vi "auto_save_settings.vi"(8 "error in":errorcluster, 10 "base path":path, 11 "all settings":T1={"Variable Settings"={"Measurement Timeout (ms)"=0}, "HSDIO Settings"={"Enable HSDIO Pulses"=TRUE, "Resource Name"="PXI1Slot6", "Clock Rate"=20000000.0, "Array of Script Triggers"=[], "Pulse Generation Script"="script script1\n     Generate RedTrap_compress_temp\nend script", "Start Trigger"={"Wait for start trigger?"=FALSE, "source (PFI 0)"="PFI0", "edge (rising)"=12, "description"=""}, "Hardware alignment quantum\n(in samples)"=1, "Inital State"="", "Idle State"="", "Active Channels"="", "Array of Waveforms"=[], "description"=""}, "DAQmx Pulse Settings"={"Enable DAQmx Pulses"=FALSE, "DAQmx Physical Channels"="", "Clock Rate"=0.0, "units/sec (ms=1000)"=0.0, "Start Trigger"={"Wait for start trigger?"=FALSE, "source"="", "edge"=0}, "Timing Sequence Control"=[]}, "DDS Settings"={"Enable DDS"=FALSE, "Array of DDS Boxes"=[]}, "Camera settings"={"Analog Gain (0-5)"=4, "Exposure Time"=0.01, "EM Gain (0-255)"=0, "Trigger Polarity"="ATP P", "External Trigger Mode"="EMD E", "Scan Speed"="SSP H", "External Trigger Source"="ESC B", "Scan Mode"="SMD N", "Super Pixel Binning\n(if enabled in Scan Mode)"="SPX 1", "Camera Sub-array acquisition region\n(if enabled in scan mode)"={"Left"=0, "Top"=0, "Width"=0, "Height"=0}, "Use camera?"=FALSE, "# image buffers"=100, "shots per measurement"=100, "Force images to U16"=FALSE, "Low Light Sensitivity"="LLS 0", "cooling"="CSW F", "fan"="FAN F", "Frame Grabber acquisition region"={"Left"=0, "Top"=0, "Right"=0, "Bottom"=0}}, "Counter Settings"={"Enable Counters"=FALSE, "Array of Counter Settings"=[]}, "Filter Cluster"={"Counter Filter thresholds"=[], "Data Filters\nROI Minimum Thresholds"=[]}, "Analog Output Parameters"={"Enable Analog Out?"=FALSE, "Physical Channel"="PXI1Slot2/ao0:2", "Minimum Value"=-10.0, "Maximum Value"=10.0, "Samples per second"=0.0, "Total AO Time (seconds)"=0.0, "Start Trigger"={"Wait for start trigger?"=FALSE, "source"="/Dev1/PFI0", "edge"=10280}, "Analog Output Waveforms (channel, time)"=[], "Export trigger"={"Export Start Trigger?"=FALSE, "output terminal"=""}}, "Notes"="", "HP83623A Generator Settings Array"=[], "Iteration Graph Settings"={"Plot Regions"="", "Plot Shots"=""}, "PI Piezo Settings"={"Enable"=FALSE, "Array of Piezo Controllers"=[]}, "Andor settings"={"Andor Path"=path "", "Copy any Andor files"=FALSE, "Wait time before copying Andor files (ms)"=0}, "Measurement Chart Settings"={"Which regions to plot (comma separated)"="", "Which shot to plot"=0}, "HP8662A Synthesized Signal Generator Array"=[], "HP83712B Synthesized CW Generator Array"=[], "TTL input"={"Enable"=FALSE, "lines"=""}} {"HSDIO Settings"."Hardware alignment quantum\n(in samples)" min=1 step=1; "HSDIO Settings"."Array of Script Triggers"."level" items=["High Level"=34, "Low Level"=35]; "HSDIO Settings"."Array of Script Triggers"."edge" items=["Rising Edge"=12, "Falling Edge"=13]; "HSDIO Settings"."Start Trigger"."edge (rising)" items=["Rising Edge"=12, "Falling Edge"=13]; "HSDIO Settings"."Clock Rate" min=0.0 max=200000000.0 format="%.2p"; "DAQmx Pulse Settings"."Start Trigger"."edge" items=["Rising"=10280, "Falling"=10171]; "DAQmx Pulse Settings"."Clock Rate" min=0.0 max=200000000.0 format="%.2p"; "Camera settings"."Frame Grabber acquisition region"."Bottom" max=512 step=1; "Camera settings"."Frame Grabber acquisition region"."Right" max=512 step=1; "Camera settings"."Frame Grabber acquisition region"."Top" max=512 step=1; "Camera settings"."Frame Grabber acquisition region"."Left" max=512 step=1; "Camera settings"."shots per measurement" min=0 step=1; "Camera settings"."# image buffers" min=0 step=1; "Camera settings"."Camera Sub-array acquisition region\n(if enabled in scan mode)"."Height" min=16 max=512 step=16; "Camera settings"."Camera Sub-array acquisition region\n(if enabled in scan mode)"."Width" min=16 max=512 step=16; "Camera settings"."Camera Sub-array acquisition region\n(if enabled in scan mode)"."Top" max=496 step=16; "Camera settings"."Camera Sub-array acquisition region\n(if enabled in scan mode)"."Left" max=496 step=16; "Camera settings"."Analog Gain (0-5)" max=5 step=1; "Counter Settings"."Array of Counter Settings"."Binwidth (ms)" format="%0.2f"; "Analog Output Parameters"."Start Trigger"."edge" items=["Rising"=10280, "Falling"=10171]; "Analog Output Parameters"."Maximum Value" format="%0.2f"; "Analog Output Parameters"."Minimum Value" format="%0.2f"}) -> (0 "error out":errorcluster)   [LabVIEW 2013]
doc: "This .vi save all the experiment settings to autosave_settings.xml in the input directory, without any prompts. For use in autosaving all settings at the beginning of each experiment.\n\nMTL 2012 Dec 27"
uses:
  Analog_output/AO_settings.ctl
  Analog_output/Analog_Output.lvclass
  filters/filters.ctl
  Counter/Counter_Settings_Control.ctl
  Counter/Counter.lvclass
  Camera/Hamamatsu_C9100-13/camera_setup.ctl
  Camera/Hamamatsu_C9100-13/Hamamatsu_C9100-13.lvclass
  <vilib>/ni845x/ni845x.llb/ni845xControl.ctl
  DDS drivers v3/DDS_box_device_reference.ctl
  DDS drivers v3/DDS RAM mode.ctl
  DDS drivers v3/DDS_box_cluster.ctl
  DDS drivers v3/Array_of_DDS_Boxes.ctl
  DDS/DDS_Settings_Cluster.ctl
  DAQmx_pulse_out/settings.ctl
  DAQmx_pulse_out/DAQmx_pulse_out.lvclass
  <instrlib>/niHSDIO/niHSDIO.llb/niHSDIO_ctl Trigger Source Values (Ring).ctl
  <instrlib>/niHSDIO/niHSDIO.llb/niHSDIO_ctl Trigger DigEdge - Edge Values (Ring).ctl
  <instrlib>/niHSDIO/niHSDIO.llb/niHSDIO_ctl Trigger Script - trigID Values (Ring).ctl
  <instrlib>/niHSDIO/niHSDIO.llb/niHSDIO_ctl Trigger DigLvl - Level Values (Ring).ctl
  HSDIO/HSDIO_settings.ctl
  HSDIO/HSDIO.lvclass
  all_settings.ctl
  GPIB/HP83623A_RF_Generator/HP83623A_array.ctl
  GPIB/HP83623A_RF_Generator/HP83623A_RF_Generator.lvclass
  PI_piezo/settings.ctl
  PI_piezo/PI_Piezo.lvclass
  Camera/Andor/Andor_settings.ctl
  gui/measurement_graph.ctl
  GPIB/RF_Generator_settings.ctl
  GPIB/GPIB.lvclass
  GPIB/RF_Generator_settings_array.ctl
  DDS drivers v3/DDS_profile.ctl
  DDS drivers v3/DDS_channel.ctl
  DDS/DDS.lvclass
  DDS drivers v3/array_of_DDS_profiles.ctl
  DDS drivers v3/array_of_DDS_channels.ctl
  TTL_input/TTL_input_settings.ctl
  TTL_input/TTL_input.lvclass
  HSDIO/waveform.ctl
  PI_piezo/piezo_channel.ctl
  PI_piezo/piezo_controller.ctl
  GPIB/HP83623A_RF_Generator/HP83623A.ctl
  ExperimentVariables/Variable_Settings.ctl
panel:
  # "Regions of Interest -->"
  # "Shots\n   |\n  V"
  # "Counters -->"
  # "Counter\n    bins\n       |\n      V"
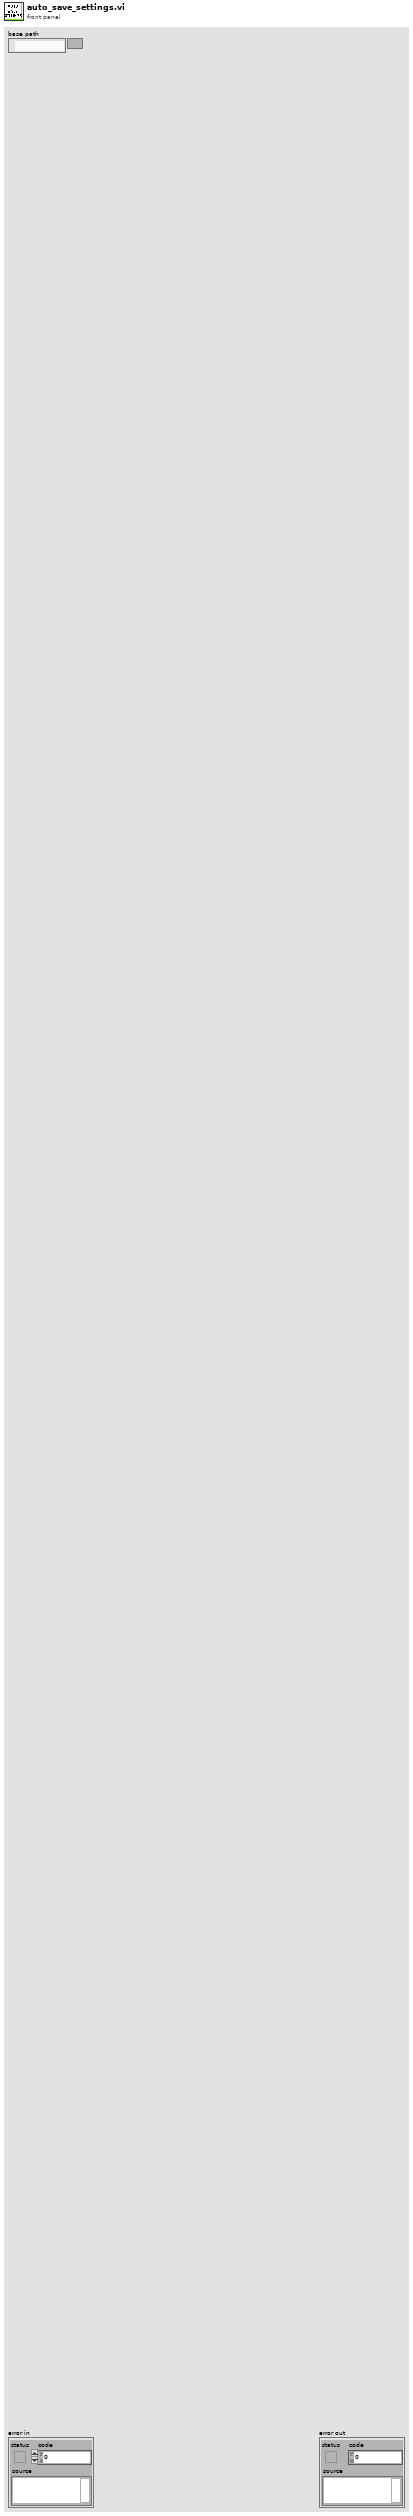
[diagram p1: front panel]
types:
  T1 = typedef "all_settings.ctl" = cluster{"Variable Settings":T2, "HSDIO Settings":T3, "DAQmx Pulse Settings":T9, "DDS Settings":T10, "Camera settings":T20, "Counter Settings":T21, "Filter Cluster":T22, "Analog Output Parameters":T23, "Notes":string, "HP83623A Generator Settings Array":T24, "Iteration Graph Settings":cluster{"Plot Regions":string, "Plot Shots":string}, "PI Piezo Settings":T26, "Andor settings":T29, "Measurement Chart Settings":T30, "HP8662A Synthesized Signal Generator Array":T31, "HP83712B Synthesized CW Generator Array":T31, "TTL input":T33}
  T2 = typedef "Variable_Settings.ctl" = cluster{"Measurement Timeout (ms)":u32}
  T3 = typedef "HSDIO.lvclass/HSDIO_settings.ctl" = cluster{"Enable HSDIO Pulses":bool, "Resource Name":refnum<k15>, "Clock Rate":dbl, "Array of Script Triggers":cluster{"trigger id (script trigger 0)":T4, "source (PFI 0)":T5, "Trigger Type":enum32{"Edge", "Level"}, "edge":T6, "level":T7}[], "Pulse Generation Script":string, "Start Trigger":cluster{"Wait for start trigger?":bool, "source (PFI 0)":T5, "edge (rising)":T6, "description":string}, "Hardware alignment quantum\n(in samples)":u16, "Inital State":string, "Idle State":string, "Active Channels":string, "Array of Waveforms":T8[], "description":string}
  T4 = typedef "niHSDIO_ctl Trigger Script - trigID Values (Ring).ctl" = string
  T5 = typedef "niHSDIO_ctl Trigger Source Values (Ring).ctl" = string
  T6 = typedef "niHSDIO_ctl Trigger DigEdge - Edge Values (Ring).ctl" = i32
  T7 = typedef "niHSDIO_ctl Trigger DigLvl - Level Values (Ring).ctl" = i32
  T8 = typedef "HSDIO.lvclass/waveform.ctl" = cluster{"name":string, "transitions":u32[], "states":u8[][]}
  T9 = typedef "DAQmx_pulse_out.lvclass/settings.ctl" = cluster{"Enable DAQmx Pulses":bool, "DAQmx Physical Channels":tag, "Clock Rate":dbl, "units/sec (ms=1000)":dbl, "Start Trigger":cluster{"Wait for start trigger?":bool, "source":tag, "edge":i32}, "Timing Sequence Control":string[][]}
  T10 = typedef "DDS_Settings_Cluster.ctl" = cluster{"Enable DDS":bool, "Array of DDS Boxes":T11}
  T11 = typedef "Array_of_DDS_Boxes.ctl" = T12[]
  T12 = typedef "DDS_box_cluster.ctl" = cluster{"DDS box device reference":T13, "Array of DDS Channels (4)":T15, "Enable":bool, "description":string}
  T13 = typedef "DDS_box_device_reference.ctl" = cluster{"NI USB-8451 device reference":T14, "DIO port":u8, "Serial Clock Rate [kHz]":u16}
  T14 = typedef "ni845xControl.ctl" = refnum<k21>
  T15 = typedef "DDS.lvclass/array_of_DDS_channels.ctl" = T16[]
  T16 = typedef "DDS.lvclass/DDS_channel.ctl" = cluster{"Power":bool, "Channel Parameters":cluster{"Ref Clock Rate [kHz]":dbl, "Full Scale Output\nPower [dBm]":dbl}, "RAM Enable":bool, "RAM Dest Type":u8, "RAM Default":cluster{"Frequency [MHz]":dbl, "Amplitude [dBm]":dbl, "Phase Offset [rad]":dbl}, "Array of DDS Profiles (8)":T17, "description":string}
  T17 = typedef "DDS.lvclass/array_of_DDS_profiles.ctl" = T18[]
  T18 = typedef "DDS_profile.ctl" = cluster{"Single Tone":cluster{"Frequency [MHz]":dbl, "Amplitude [dBm]":dbl, "Phase Offset [rad]":dbl}, "RAM Mode ":T19, "Zero-crossing":bool, "No Dwell High":bool, "Function/Static":bool, "RAM Function Settings":string[], "RAM Static Array":dbl[], "description":string}
  T19 = typedef "DDS RAM mode.ctl" = enum16{"Direct Switch", "Ramp Up", "Bidirectional Ramp", "Continuous Bidirectional Ramp", "Continuous Recirculate", "Direct Switch 2", "Direct Switch 3", "Direct Switch 4"}
  T20 = typedef "Hamamatsu_C9100-13.lvclass/camera_setup.ctl" = cluster{"Analog Gain (0-5)":u8, "Exposure Time":dbl, "EM Gain (0-255)":u8, "Trigger Polarity":string, "External Trigger Mode":string, "Scan Speed":string, "External Trigger Source":string, "Scan Mode":string, "Super Pixel Binning\n(if enabled in Scan Mode)":string, "Camera Sub-array acquisition region\n(if enabled in scan mode)":cluster{"Left":u16, "Top":u16, "Width":u16, "Height":u16}, "Use camera?":bool, "# image buffers":i32, "shots per measurement":i32, "Force images to U16":bool, "Low Light Sensitivity":string, "cooling":string, "fan":string, "Frame Grabber acquisition region":cluster{"Left":i32, "Top":i32, "Right":i32, "Bottom":i32}}
  T21 = typedef "Counter.lvclass/Counter_Settings_Control.ctl" = cluster{"Enable Counters":bool, "Array of Counter Settings":cluster{"Counter Channel":tag, "Time-Bin Clock Channel":tag, "Binwidth (ms)":dbl}[]}
  T22 = typedef "filters.ctl" = cluster{"Counter Filter thresholds":u32[][], "Data Filters\nROI Minimum Thresholds":u64[][]}
  T23 = typedef "Analog_Output.lvclass/AO_settings.ctl" = cluster{"Enable Analog Out?":bool, "Physical Channel":tag, "Minimum Value":dbl, "Maximum Value":dbl, "Samples per second":dbl, "Total AO Time (seconds)":dbl, "Start Trigger":cluster{"Wait for start trigger?":bool, "source":tag, "edge":i32}, "Analog Output Waveforms (channel, time)":dbl[][], "Export trigger":cluster{"Export Start Trigger?":bool, "output terminal":tag}}
  T24 = typedef "HP83623A_RF_Generator.lvclass/HP83623A_array.ctl" = T25[]
  T25 = typedef "HP83623A_RF_Generator.lvclass/HP83623A.ctl" = cluster{"Frequency (Hz)":dbl, "Power (dBm)":dbl, "Enabled":bool, "initialized":bool, "RF Output On/Off":bool, "External Trigger?":bool, "VISA Session":refnum<visa-resource-name>, "Generator Name":string}
  T26 = typedef "PI_Piezo.lvclass/settings.ctl" = cluster{"Enable":bool, "Array of Piezo Controllers":T27[]}
  T27 = typedef "PI_Piezo.lvclass/piezo_controller.ctl" = cluster{"Enable":bool, "Serial No.":string, "Array of Piezo Channels":T28[]}
  T28 = typedef "PI_Piezo.lvclass/piezo_channel.ctl" = cluster{"Servo":bool, "Set Position":dbl}
  T29 = typedef "Andor_settings.ctl" = cluster{"Andor Path":path, "Copy any Andor files":bool, "Wait time before copying Andor files (ms)":u16}
  T30 = typedef "measurement_graph.ctl" = cluster{"Which regions to plot (comma separated)":string, "Which shot to plot":u8}
  T31 = typedef "GPIB.lvclass/RF_Generator_settings_array.ctl" = T32[]
  T32 = typedef "GPIB.lvclass/RF_Generator_settings.ctl" = cluster{"Enable":bool, "Description":string, "GPIB channel #":u8, "Frequency (MHz)":dbl, "Power (dBm)":dbl}
  T33 = typedef "TTL_input.lvclass/TTL_input_settings.ctl" = cluster{"Enable":bool, "lines":tag}
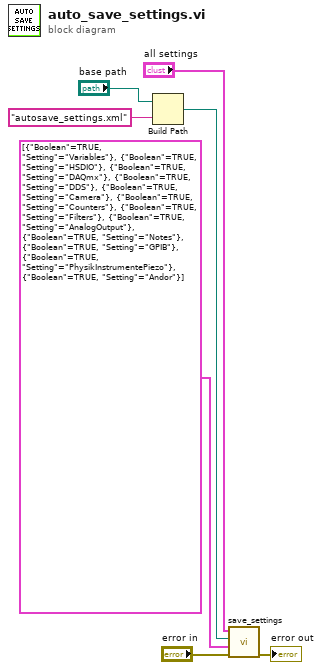
[diagram p0: block diagram]
diagram:
  n1 = Build Path(base path="base path", name or relative path="autosave_settings.xml" ("time format string (%c)")) -> (appended path=w1:path)
  n2 = call "save_settings.vi"("error in"="error in", "Which settings to save"=cluster{"Boolean":bool, "Setting":string}[] [{"Boolean"=TRUE, "Setting"="Variables"}, {"Boolean"=TRUE, "Setting"="HSDIO"}, {"Boolean"=TRUE, "Setting"="DAQmx"}, {"Boolean"=TRUE, "Setting"="DDS"}, {"Boolean"=TRUE, "Setting"="Camera"}, {"Boolean"=TRUE, "Setting"="Counters"}, {"Boolean"=TRUE, "Setting"="Filters"}, {"Boolean"=TRUE, "Setting"="AnalogOutput"}, {"Boolean"=TRUE, "Setting"="Notes"}, {"Boolean"=TRUE, "Setting"="GPIB"}, {"Boolean"=TRUE, "Setting"="PhysikInstrumentePiezo"}, {"Boolean"=TRUE, "Setting"="Andor"}], "XML File Path"=w1, "all settings"="all settings") -> ("error out"=→"error out":errorcluster)  [unwired: 7 in]
